vi "DSE1_x_defaut.vi"(1 "p_LN":T1) -> (0 "X-LN (Défaut)":T2)   [LabVIEW 2010, in "lv_02.lvlib"]
uses:
  lv_01/do_serie-c.ctl
  p_5E1_LN.ctl
  lv_01/0002-03.vi
  lv_02.lvlib
  lv_01/lv_01.lvlib
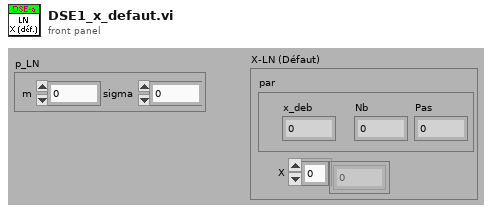
[diagram p1: front panel]
types:
  T1 = typedef "lv_02.lvlib/p_5E1_LN.ctl" = cluster{"m":dbl, "sigma":dbl}
  T2 = typedef "lv_01.lvlib/do_serie-c.ctl" = cluster{"X":dbl[], "par":cluster{"x_deb":dbl, "Pas":dbl, "Nb":dbl}}
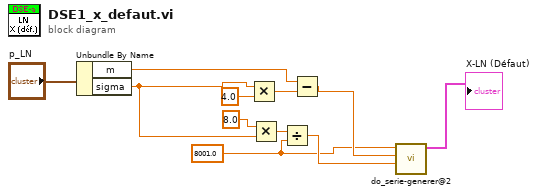
[diagram p0: block diagram]
diagram:
  w1 = 8001.0 ("y")
  n1 = Unbundle By Name("p_LN") -> ("m"=w6:dbl, "sigma"=w7:dbl)
  n2 = Multiply(x=w7, y=4.0) -> (x*y=w8:dbl)
  n3 = Multiply(x=8.0, y=w7) -> (x*y=w11:dbl)
  n4 = Divide(x=w11, y=w1) -> (x/y=w3:dbl)
  n5 = Subtract(x=w6, y=w8) -> (x-y=w4:dbl)
  n6 = call-poly "do_serie-generer@2.vi"("Pas"=w3, "x_deb"=w4, "Nb"=w1) -> ("sér. (s)"=→"X-LN (Défaut)":T2)  [unwired: 8 in]
